vi "Script New Cases in Case Structure.vi"() -> ()   [LabVIEW 2020]
panel:
  out "error out":errorcluster
  in  "vi path":path
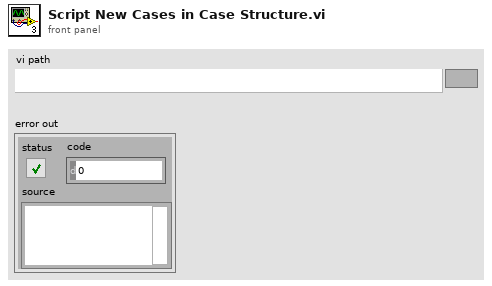
[diagram p1: front panel]
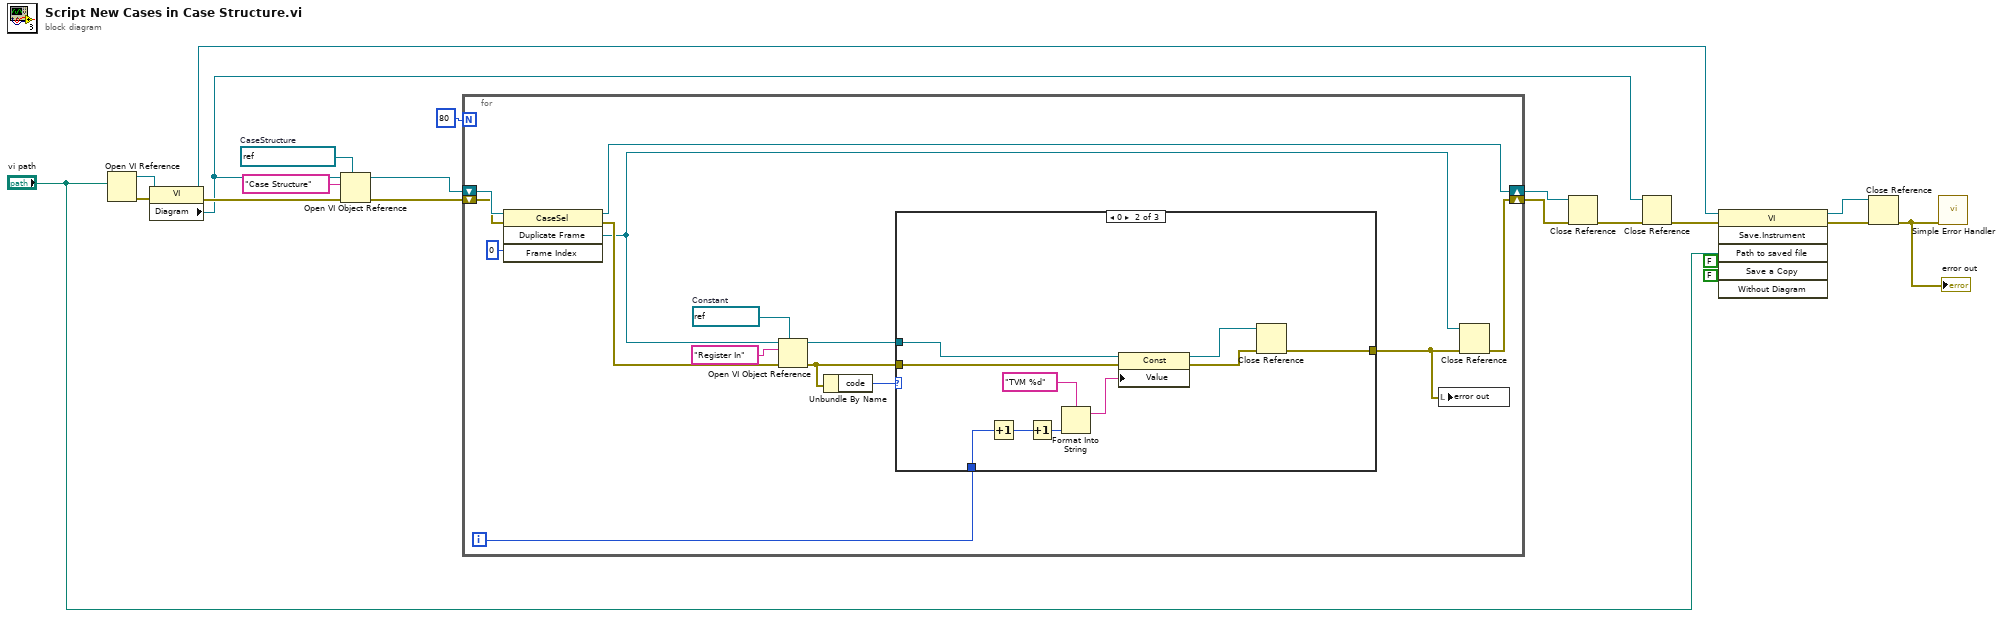
[diagram p0: block diagram]
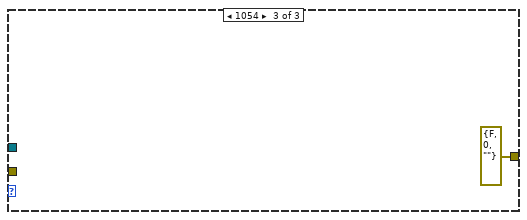
[diagram p3: hidden frame]
diagram:
  w19 = refnum<vi> refnum  # CaseStructure
  n1 = Open VI Reference(vi path="vi path") -> (vi reference=w20:refnum<vi>, error out=w12:errorcluster)  [unwired: 5 in]
  n2 = property class="VI"(reference=w20, error in=w12) -> (reference out=w13:refnum<vi>, error out=w11:errorcluster, "Diagram"=w1:refnum<vi>)
  n3 = Open VI Object Reference(7:w19, 8:w11, 10:"Case Structure" ("Case Structure Label"), 11:w1) -> (0:w10:errorcluster, 3:w18:refnum<vi>)
  n4 = for {
    N: 80 -> [_]
    shift-right: [w29] -> w7
    shift-left: w10 -> [w32]
    shift-right: [w27] -> w8
    shift-left: w18 -> [w34]
    i -> [w31]
    w24 = refnum<vi> refnum  # Constant
    n5 = invoke class="CaseSel" method="Duplicate Frame"(reference=w34, error in=w32, "Frame Index"=u32 0) -> (reference out=w27:refnum<vi>, error out=w30:errorcluster, "Duplicate Frame"=w26:refnum<vi>)  [unwired: 1 in, 1 out]
    n6 = Open VI Object Reference(7:w24, 8:w30, 10:"Register In" ("Case Structure Label"), 11:w26) -> (0:w22:errorcluster, 3:w23:refnum<vi>)
    n7 = Unbundle By Name(w22) -> ("code"=w21:i32)
    n8 = case shown="0" w21 {
      tunnel: w31 -> [_ w45 _]
      tunnel: [w35 w44 errorcluster {"status"=FALSE, "code"=0, "source"=""} ("error out")] -> w28
      tunnel: w23 -> [_ w40 _]
      tunnel: w22 -> [w35 w39 _]
      frame Default {
      }
      frame 0 {
        n9 = Increment(x=w45) -> (x+1=w36:i32)
        n10 = Increment(x=w36) -> (x+1=w42:i32)
        n11 = Format Into String(format string="TVM %d", w42) -> (resulting string=w43:string)  [unwired: 2 in, 1 out]
        n12 = property class="Const"(reference=w40, error in=w39, "Value"=w43) -> (reference out=w38:refnum<vi>, error out=w37:errorcluster)
        n13 = Close Reference(reference=w38, error in (no error)=w37) -> (error out=w44:errorcluster)
      }
      frame 1054 {
      }
    }
    n14 = local write "error out"(w28) -> ()
    n15 = Close Reference(reference=w26, error in (no error)=w28) -> (error out=w29:errorcluster)
  }
  n16 = Close Reference(reference=w8, error in (no error)=w7) -> (error out=w3:errorcluster)
  n17 = Close Reference(reference=w1, error in (no error)=w3) -> (error out=w2:errorcluster)
  n18 = invoke class="VI" method="Save.Instrument"(reference=w13, error in=w2, "Path to saved file"="vi path", "Save a Copy"=FALSE, "Without Diagram"=FALSE) -> (reference out=w5:refnum<vi>, error out=w6:errorcluster)  [unwired: 1 in, 4 out]
  n19 = Close Reference(reference=w5, error in (no error)=w6) -> (error out=w4:errorcluster)
  "error out" <- w4
  n20 = call <vilib>:"Simple Error Handler.vi"("error in (no error)"=w4) -> ()  [unwired: 4 in, 5 out]
